vi "Drive Status FGV.vi"(8 "error in":errorcluster, 9 "Disconnect Drive":bool, 10 "Connect Drive":bool, 11 "Enum":enum16{"Read", "Write"}(ring)) -> (0 "error out":errorcluster, 1 "Disconnect Drive out":bool, 2 "Connect Drive Out":bool)   [LabVIEW 2022 SP3]
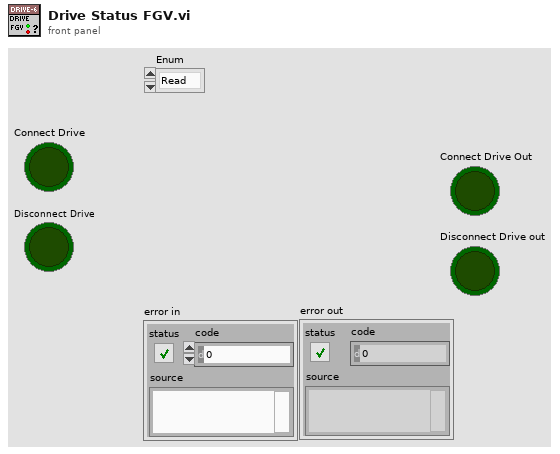
[diagram p1: front panel]
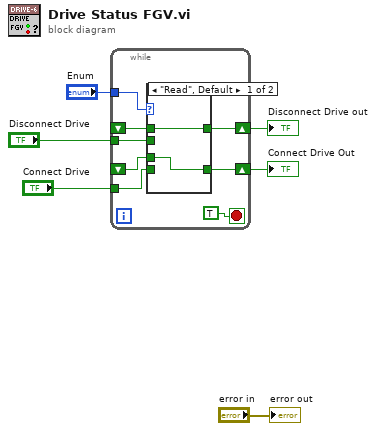
[diagram p0: block diagram]
diagram:
  n1 = while {
    tunnel: "Enum" -> [w14]
    tunnel: "Connect Drive" -> [w12]
    shift-right: [w11] -> w3
    shift-left: _ -> [w10]
    tunnel: "Disconnect Drive" -> [w9]
    shift-right: [w8] -> w1
    shift-left: _ -> [w7]
    stop <- TRUE stop-if-true
    n2 = case shown="\"Read\", Default" w14 {
      tunnel: w12 -> [_ w18]
      tunnel: [w16 w18] -> w11
      tunnel: w10 -> [w16 _]
      tunnel: w9 -> [_ w17]
      tunnel: [w15 w17] -> w8
      tunnel: w7 -> [w15 _]
      frame "Read", Default {
      }
      frame "Write" {
      }
    }
  }
  "Connect Drive Out" <- w3
  "Disconnect Drive out" <- w1
  "error out" <- "error in"
